vi "Demo.vi"() -> ()   [LabVIEW 2009]
panel:
  in  "Initial additional data":i32(slide)=44 scale=0.0..800.0
  in  "Real time":bool=TRUE
  out "Graph of input space (2 inputs = 2 dimensions) real time":T1(graph)
  in  "Number of hidden neurons":i32(slide)=10 scale=0.0..20.0
  in  "Comments":string="Training is done on the neural network below with the initial training data A and B. After the network learns the classes of the initial data, more data is introduced and the neural network will classify them."
  in  "stop":bool
  out "Error":dbl(graph)
  in  "Learning Rate":dbl(slide)=0.336734693877551 scale=0.0..1.0
  out "Graph of input space (2 inputs = 2 dimensions) end result":T1(graph)
  in  "B":dbl[][](array[slide])=[[2.040816326530612, -1.959183673469388], [1.3061224489795915, -1.959183673469388], [1.6326530612244894, -1.142857142857143], [-2.285714285714286, 2.285714285714285], [0.8163265306122445, -1.306122448979592], [-1.959183673469388, 1.3061224489795915], [-1.306122448979592, 1.6326530612244894], [1.9591836734693873, 1.9591836734693873], [2.5306122448979584, 1.7959183673469383]] scale=-4.0..4.0
  in  "A":dbl[][](array[slide])=[[-0.0816326530612248, -3.191891195797325e-16], [2.040816326530612, -3.191891195797325e-16], [2.2040816326530606, -0.24489795918367377], [-1.7142857142857144, -2.285714285714286], [-2.2040816326530615, -1.3877551020408165], [-1.795918367346939, -0.4897959183673472], [-1.3877551020408165, -1.795918367346939], [0.0, 2.285714285714285], [0.4081632653061221, 1.7959183673469383]] scale=-4.0..4.0
  # "Artificial Neural Network Example"
  # "Classify 2 dimensional objects a with A and b with B"
  # "Initial training data"
  # "Training set"
  # "2 input neurons"
  # "2 output neurons"
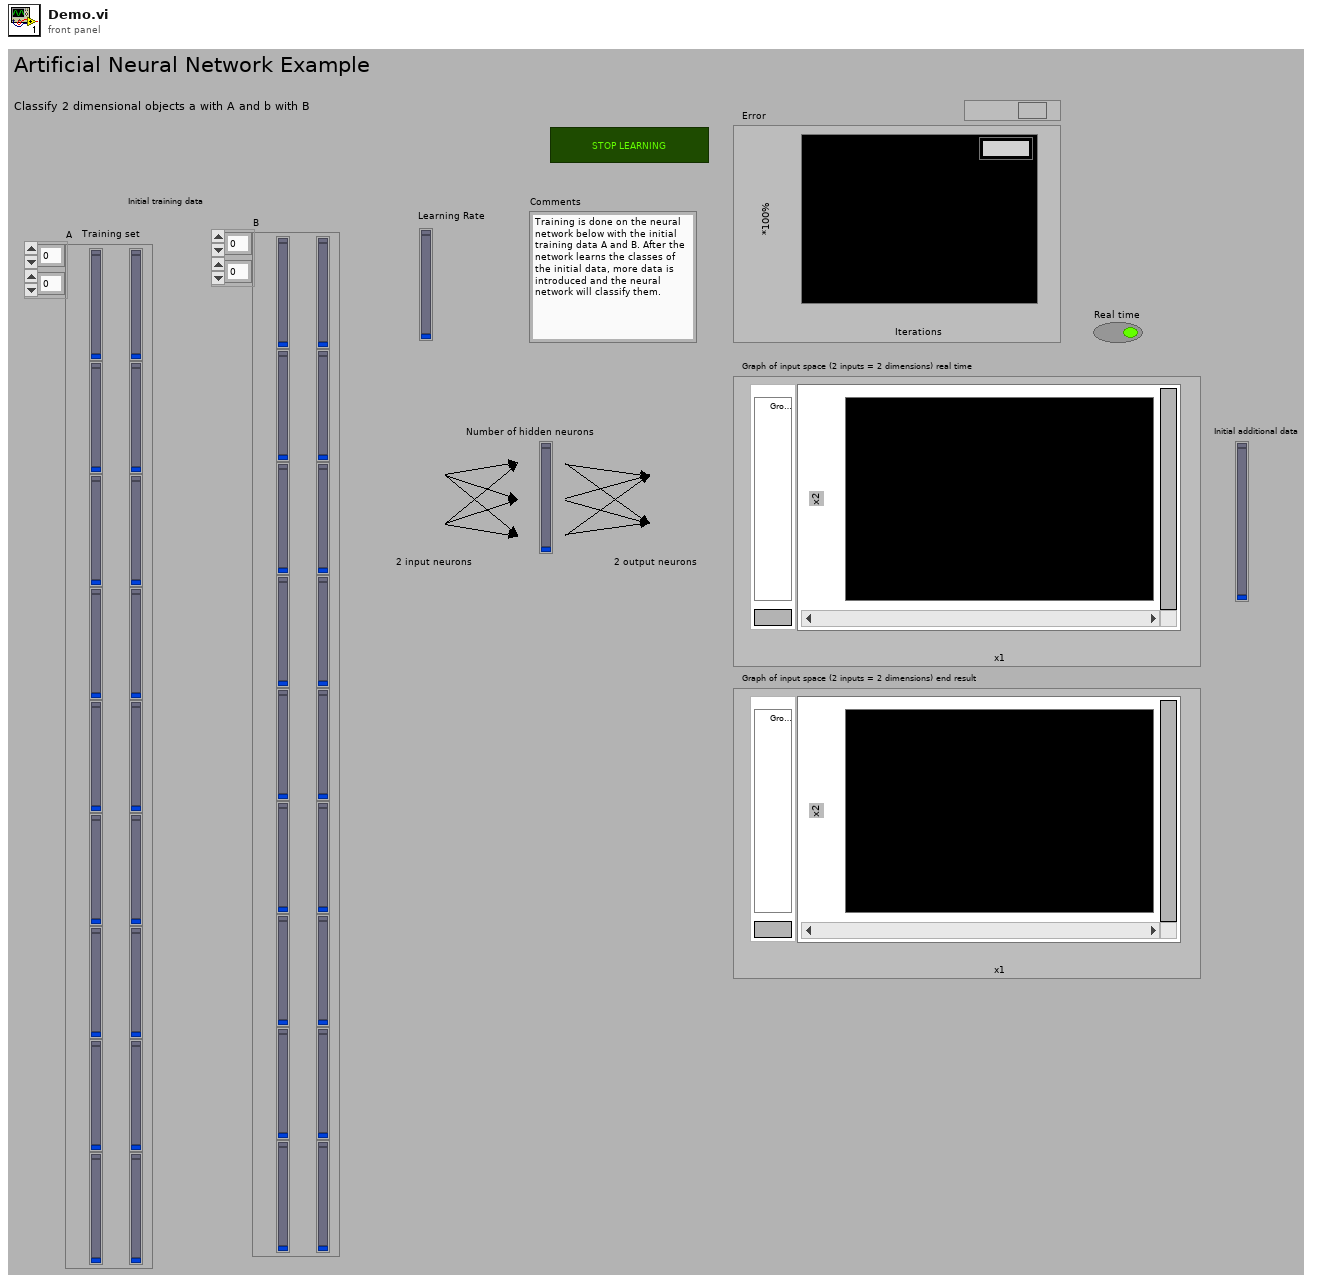
[diagram p1: front panel]
types:
  T1 = cluster{cluster{"A":dbl[], "A":dbl[]}, cluster{"B":dbl[], "B":dbl[]}}
  T2 = cluster{cluster{dbl[], dbl[]}, cluster{dbl[], dbl[]}}
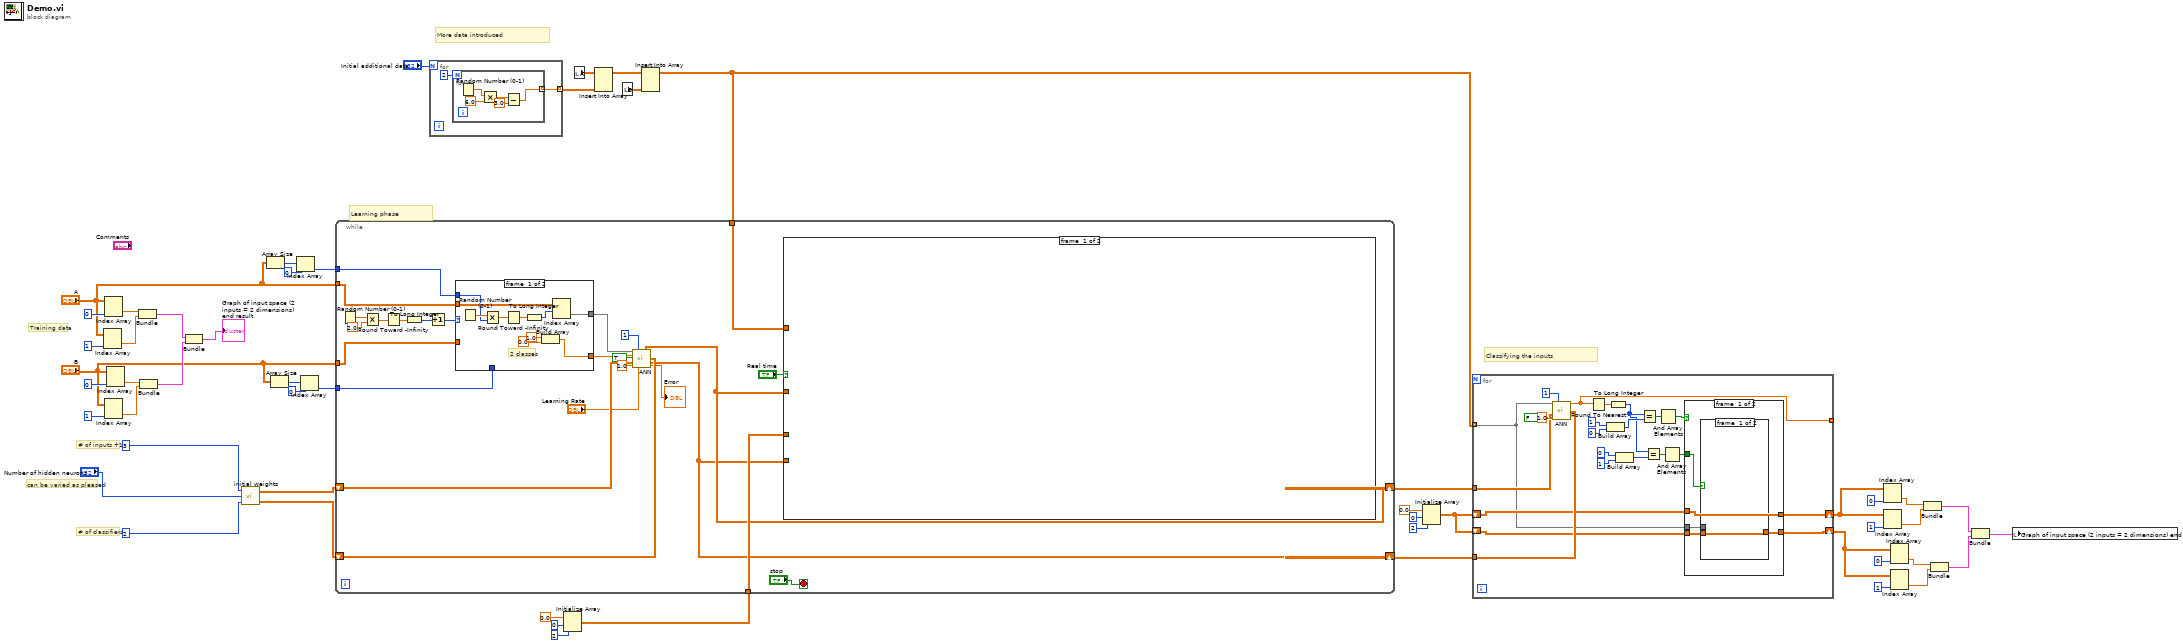
[diagram p0: block diagram]
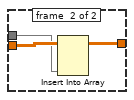
[diagram p2: hidden frame]
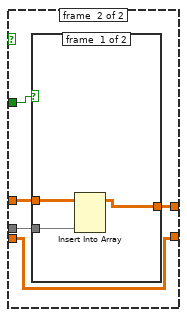
[diagram p3: hidden frame]
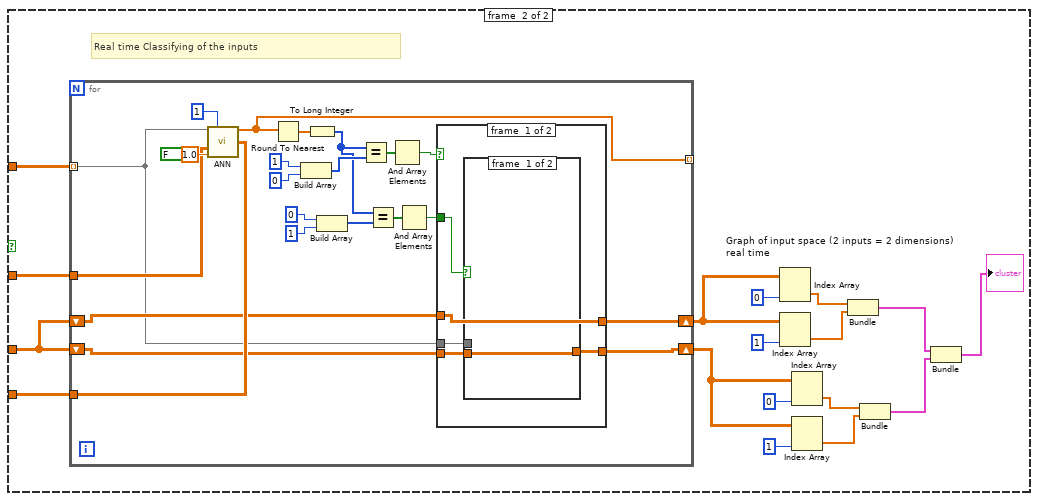
[diagram p5: hidden frame]
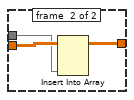
[diagram p6: hidden frame]
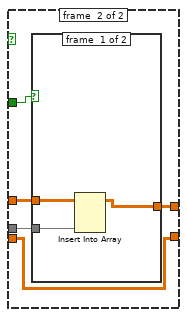
[diagram p7: hidden frame]
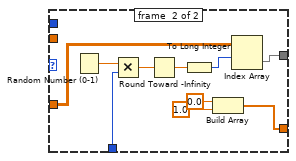
[diagram p9: hidden frame]
diagram:
  # "Classifying the inputs"
  # "More data introduced"
  # "can be varied as pleased"
  # "Training data"
  # "Learning phase"
  # "# of inputs +1"
  # "# of classifiers"
  n1 = Index Array(array="A", index (col)=1 ("index (row)")) -> (element=w46:dbl[])  [unwired: 1 in]
  n2 = Index Array(array="A", index (col)=0 ("index (row)")) -> (element=w47:dbl[])  [unwired: 1 in]
  n3 = Index Array(array="B", index (col)=1 ("index (row)")) -> (element=w50:dbl[])  [unwired: 1 in]
  n4 = Index Array(array="B", index (col)=0 ("index (row)")) -> (element=w52:dbl[])  [unwired: 1 in]
  n5 = Bundle("A"=w47, "A"=w46) -> (w44:cluster{"A":dbl[], "A":dbl[]})  [unwired: 1 in]
  n6 = Bundle("B"=w52, "B"=w50) -> (w43:cluster{"B":dbl[], "B":dbl[]})  [unwired: 1 in]
  n7 = Bundle(w44, w43) -> (→"Graph of input space (2 inputs = 2 dimensions) end result":T1)  [unwired: 1 in]
  n8 = call "initial weights.vi"("Number of classifiers"=2, "Number of hidden neurons"="Number of hidden neurons", "Inputs + 1"=3) -> ("Weights 2"=w36:dbl[][], "Weights 1"=w37:dbl[][])
  n9 = Array Size(array="A") -> (size(s)=w42:i32[])
  n10 = Array Size(array="B") -> (size(s)=w35:i32[])
  n11 = Index Array(array=w42, index=0) -> (element=w40:i32)
  n12 = Index Array(array=w35, index=0) -> (element=w33:i32)
  n13 = for {
    N: "Initial additional data" -> [_]
    tunnel: [w55] -> w30 mode=indexing
    n14 = for {
      N: 2 -> [_]
      tunnel: [w56] -> w55 mode=indexing
      n15 = Random Number (0-1)() -> (number: 0 to 1=w60:dbl)
      n16 = Multiply(x=w60, y=6.0) -> (x*y=w58:dbl)
      n17 = Subtract(x=w58, y=3.0) -> (x-y=w56:dbl)
    }
  }
  n18 = Initialize Array(0.0 ("element"), 0 ("dimension size"), 2 ("dimension size")) -> (w2:dbl[][])
  n19 = local read "A"() -> (w25:dbl[][])
  n20 = Insert Into Array(array=w25, new element=w30) -> (w28:dbl[][])  [unwired: 2 in]
  n21 = local read "B"() -> (w1:dbl[][])
  n22 = Insert Into Array(array=w28, new element=w1) -> (w3:dbl[][])  [unwired: 2 in]
  n23 = while {
    tunnel: "A" -> [w81]
    tunnel: "B" -> [w80]
    tunnel: w40 -> [w79]
    shift-right: [w64] -> w24
    shift-left: w37 -> [w74]
    shift-right: [w63] -> w23
    shift-left: w36 -> [w73]
    tunnel: w33 -> [w75]
    tunnel: w3 -> [w65]
    tunnel: w2 -> [w66]
    stop <- "stop" stop-if-true
    n24 = Random Number (0-1)() -> (number: 0 to 1=w85:dbl)
    n25 = Multiply(x=w85, y=2.0) -> (x*y=w83:dbl)
    n26 = Round Toward -Infinity(1:w83) -> (0:w82:dbl)
    n27 = To Long Integer(number=w82) -> (32bit integer=w68:i32)
    n28 = Increment(x=w68) -> (x+1=w67:i32)
    n29 = case shown="1, Default" w67 {
      tunnel: w81 -> [w153 _]
      tunnel: w80 -> [_ w157]
      tunnel: w79 -> [w149 _]
      tunnel: [w147 w155] -> w76
      tunnel: [w144 w154] -> w77
      tunnel: w75 -> [_ w156]
      frame #0 {
        # "2 classes"
        n30 = Random Number (0-1)() -> (number: 0 to 1=w152:dbl)
        n31 = Multiply(x=w152, y=w149) -> (x*y=w151:dbl)
        n32 = Round Toward -Infinity(1:w151) -> (0:w150:dbl)
        n33 = To Long Integer(number=w150) -> (32bit integer=w148:i32)
        n34 = Build Array(1.0 ("element"), 0.0 ("element")) -> (w144:dbl[])
        n35 = Index Array(array=w153, index (row)=w148) -> (element=w147:dbl[])  [unwired: 1 in]
      }
      frame #1 {
        n36 = Random Number (0-1)() -> (number: 0 to 1=w158:dbl)
        n37 = Multiply(x=w158, y=w156) -> (x*y=w159:dbl)
        n38 = Round Toward -Infinity(1:w159) -> (0:w160:dbl)
        n39 = To Long Integer(number=w160) -> (32bit integer=w161:i32)
        n40 = Build Array(0.0 ("element"), 1.0 ("element")) -> (w154:dbl[])
        n41 = Index Array(array=w157, index (row)=w161) -> (element=w155:dbl[])  [unwired: 1 in]
      }
    }
    n42 = call "ANN.vi"("Input"=w76, "Iterations"=1, "Beta"=1.0, "Target Output"=w77, "Weight_2"=w73, "Weight_1"=w74, "Back Propagation"=TRUE, "Learning Rate"="Learning Rate") -> ("Weight_2_out"=w63:dbl[][], "Weight_1_out"=w64:dbl[][], "Error"=→"Error":dbl)  [unwired: 4 in, 1 out]
    n43 = case shown="True" "Real time" {
      tunnel: w66 -> [_ w90]
      tunnel: w65 -> [_ w89]
      tunnel: w64 -> [_ w88]
      tunnel: w63 -> [_ w87]
      frame #0 {
      }
      frame #1 {
        # "Real time Classifying of the inputs"
        n44 = for {
          tunnel: w89 -> [w108] mode=indexing
          tunnel: w88 -> [w123]
          tunnel: w87 -> [w122]
          shift-right: [w107] -> w100
          shift-left: w90 -> [w109]
          shift-right: [w105] -> w93
          shift-left: w90 -> [w106]
          tunnel: [w104] -> _ mode=indexing
          n45 = call "ANN.vi"("Input"=w108, "Iterations"=1, "Beta"=1.0, "Weight_2"=w122, "Weight_1"=w123, "Back Propagation"=FALSE) -> ("output"=w104:dbl[])  [unwired: 6 in, 3 out]
          n46 = Round To Nearest(number=w104) -> (nearest integer value=w121:dbl[])
          n47 = Build Array(1, 0) -> (w118:i32[])
          n48 = To Long Integer(number=w121) -> (32bit integer=w112:i32[])
          n49 = Build Array(0, 1) -> (w113:i32[])
          n50 = Equal?(x=w112, y=w118) -> (x = y?=w117:bool[])
          n51 = Equal?(x=w112, y=w113) -> (x = y?=w111:bool[])
          n52 = And Array Elements(Boolean array=w117) -> (logical AND=w116:bool)
          n53 = And Array Elements(Boolean array=w111) -> (logical AND=w110:bool)
          n54 = case shown="False" w116 {
            tunnel: w110 -> [w126 w139]
            tunnel: w109 -> [w130 w138]
            tunnel: w108 -> [w128 w137]
            tunnel: [w130 w136] -> w107
            tunnel: w106 -> [w129 w135]
            tunnel: [w127 w135] -> w105
            frame #0 {
              n55 = case shown="False" w126 {
                tunnel: w129 -> [w131 w134]
                tunnel: w128 -> [_ w133]
                tunnel: [w131 w132] -> w127
                frame #0 {
                }
                frame #1 {
                  n56 = Insert Into Array(array=w134, new element=w133) -> (w132:dbl[][])  [unwired: 2 in]
                }
              }
            }
            frame #1 {
              n57 = case shown="False" w139 {
                tunnel: w138 -> [w142 w143]
                tunnel: w137 -> [w141 _]
                tunnel: [w140 w143] -> w136
                frame #0 {
                  n58 = Insert Into Array(array=w142, new element=w141) -> (w140:dbl[][])  [unwired: 2 in]
                }
                frame #1 {
                }
              }
            }
          }
        }
        n59 = Index Array(array=w100, index (col)=0 ("index (row)")) -> (element=w99:dbl[])  [unwired: 1 in]
        n60 = Index Array(array=w100, index (col)=1 ("index (row)")) -> (element=w98:dbl[])  [unwired: 1 in]
        n61 = Index Array(array=w93, index (col)=0 ("index (row)")) -> (element=w95:dbl[])  [unwired: 1 in]
        n62 = Index Array(array=w93, index (col)=1 ("index (row)")) -> (element=w94:dbl[])  [unwired: 1 in]
        n63 = Bundle(w99, w98) -> (w91:cluster{dbl[], dbl[]})  [unwired: 1 in]
        n64 = Bundle(w95, w94) -> (w92:cluster{dbl[], dbl[]})  [unwired: 1 in]
        n65 = Bundle(w91, w92) -> (→"Graph of input space (2 inputs = 2 dimensions) real time":T2)  [unwired: 1 in]
      }
    }
  }
  n66 = Initialize Array(0.0 ("element"), 0 ("dimension size"), 2 ("dimension size")) -> (w19:dbl[][])
  n67 = for {
    tunnel: w3 -> [w169] mode=indexing
    tunnel: w24 -> [w184]
    tunnel: w23 -> [w183]
    shift-right: [w168] -> w18
    shift-left: w19 -> [w170]
    shift-right: [w166] -> w11
    shift-left: w19 -> [w167]
    tunnel: [w165] -> _ mode=indexing
    n68 = call "ANN.vi"("Input"=w169, "Iterations"=1, "Beta"=1.0, "Weight_2"=w183, "Weight_1"=w184, "Back Propagation"=FALSE) -> ("output"=w165:dbl[])  [unwired: 6 in, 3 out]
    n69 = Round To Nearest(number=w165) -> (nearest integer value=w182:dbl[])
    n70 = Build Array(1, 0) -> (w179:i32[])
    n71 = To Long Integer(number=w182) -> (32bit integer=w173:i32[])
    n72 = Build Array(0, 1) -> (w174:i32[])
    n73 = Equal?(x=w173, y=w179) -> (x = y?=w178:bool[])
    n74 = Equal?(x=w173, y=w174) -> (x = y?=w172:bool[])
    n75 = And Array Elements(Boolean array=w178) -> (logical AND=w177:bool)
    n76 = And Array Elements(Boolean array=w172) -> (logical AND=w171:bool)
    n77 = case shown="True" w177 {
      tunnel: w171 -> [w187 w200]
      tunnel: w170 -> [w191 w199]
      tunnel: w169 -> [w189 w198]
      tunnel: [w191 w197] -> w168
      tunnel: w167 -> [w190 w196]
      tunnel: [w188 w196] -> w166
      frame #0 {
        n78 = case shown="True" w187 {
          tunnel: w190 -> [w192 w195]
          tunnel: w189 -> [_ w194]
          tunnel: [w192 w193] -> w188
          frame #0 {
          }
          frame #1 {
            n79 = Insert Into Array(array=w195, new element=w194) -> (w193:dbl[][])  [unwired: 2 in]
          }
        }
      }
      frame #1 {
        n80 = case shown="False" w200 {
          tunnel: w199 -> [w203 w204]
          tunnel: w198 -> [w202 _]
          tunnel: [w201 w204] -> w197
          frame #0 {
            n81 = Insert Into Array(array=w203, new element=w202) -> (w201:dbl[][])  [unwired: 2 in]
          }
          frame #1 {
          }
        }
      }
    }
  }
  n82 = Index Array(array=w18, index (col)=0 ("index (row)")) -> (element=w17:dbl[])  [unwired: 1 in]
  n83 = Index Array(array=w18, index (col)=1 ("index (row)")) -> (element=w16:dbl[])  [unwired: 1 in]
  n84 = Index Array(array=w11, index (col)=0 ("index (row)")) -> (element=w13:dbl[])  [unwired: 1 in]
  n85 = Index Array(array=w11, index (col)=1 ("index (row)")) -> (element=w12:dbl[])  [unwired: 1 in]
  n86 = Bundle(w17, w16) -> (w9:cluster{dbl[], dbl[]})  [unwired: 1 in]
  n87 = Bundle(w13, w12) -> (w10:cluster{dbl[], dbl[]})  [unwired: 1 in]
  n88 = Bundle(w9, w10) -> (w8:T2)  [unwired: 1 in]
  n89 = local write "Graph of input space (2 inputs = 2 dimensions) end result"(w8) -> ()
